vi "tcsWEP_getEvent_wavefrontError.vi"(8 "error in (no error)":errorcluster, 11 "logevent_wavefrontError_Ctl":T1={"sensorId"=0, "annularZernikePoly[19]"=[0.0, 0.0, 0.0, 0.0, 0.0, 0.0, 0.0, 0.0, 0.0, 0.0, 0.0, 0.0, 0.0, 0.0, 0.0, 0.0, 0.0, 0.0, 0.0], "timestamp"=0.0, "priority"=0}) -> (0 "error out":errorcluster, 2 "function return":i32, 3 "logevent_wavefrontError_Ctl out":T1)   [LabVIEW 2016, in "SALLV_tcsWEP.lvlib"]
doc: "int tcsWEP_shm_getEvent_wavefrontErrorLV(tcsWEP_logevent_wavefrontErrorLV *logevent_wavefrontError_Ctl );"
uses:
  SALLV_tcsWEP.lvlib
  DataTypes/logevent_wavefrontError.ctl
  SALLV_tcsWEP.so
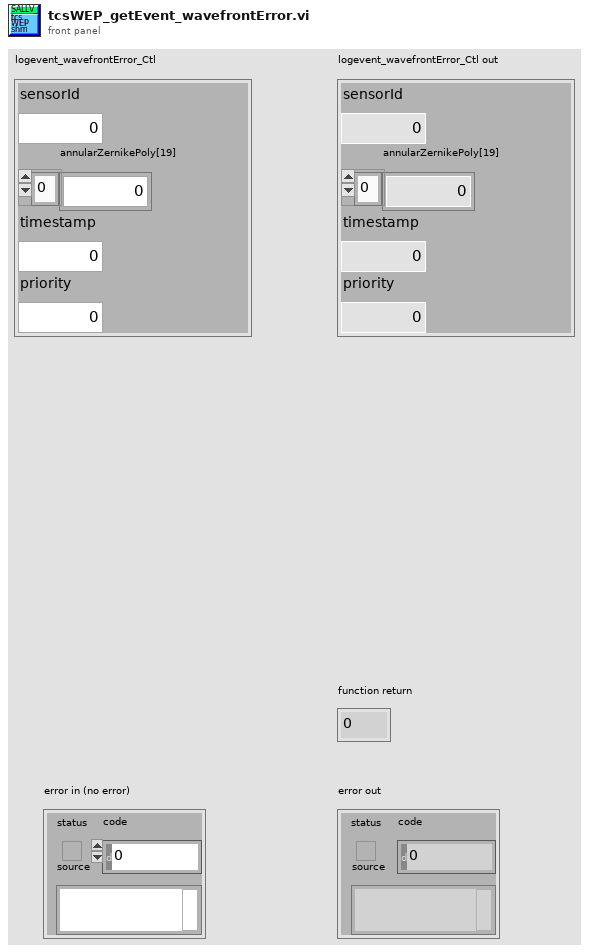
[diagram p1: front panel]
types:
  T1 = typedef "SALLV_tcsWEP.lvlib/logevent_wavefrontError.ctl" = cluster{"sensorId":i16, "annularZernikePoly[19]":dbl[], "timestamp":dbl, "priority":i32}
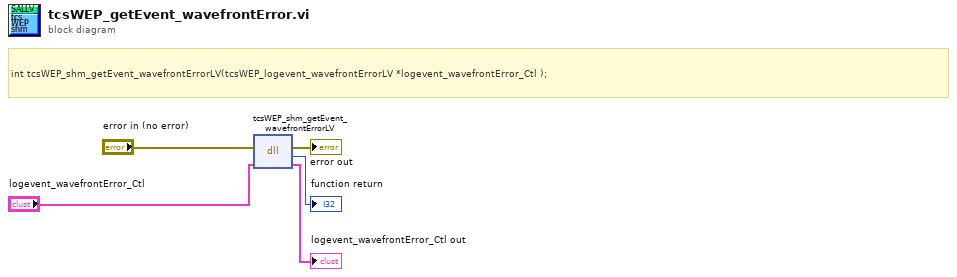
[diagram p0: block diagram]
diagram:
  # "int tcsWEP_shm_getEvent_wavefrontErrorLV(tcsWEP_logevent_wavefrontErrorLV *logevent_wavefrontError_Ctl );"
  n1 = dll-call lib="home/ttsai/Documents/salAPI/SALLV_tcsWEP.*" fn="tcsWEP_shm_getEvent_wavefrontErrorLV"(error in="error in (no error)", "logevent_wavefrontError_Ctl"="logevent_wavefrontError_Ctl") -> (error out=→"error out":errorcluster, →"function return":i32, "logevent_wavefrontError_Ctl"=→"logevent_wavefrontError_Ctl out":T1)  [unwired: 2 in, 1 out]
